vi "Read Measurement.vi"(8 "Error In (no error)":errorcluster, 10 "Value Selection (0: X)":u16(ring) items=["X", "Y", "R [V]", "R [dBm]", "Phi", "CH1 Display", "CH2 Display", "AUX 1", "AUX 2"], 11 "VISA Resource Name":refnum<visa-resource-name>) -> (0 "Error Out":errorcluster, 2 "Value":dbl format="%.2e", 3 "VISA Resource Name Out":refnum<visa-resource-name>)   [LabVIEW 2010, in "Stanford Research 844.lvlib"]
doc: "This VI measures one of parameter's values."
uses:
  <instrlib>/Stanford Research 844/Stanford Research 844.lvlib
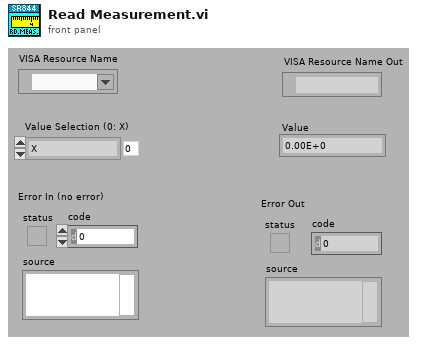
[diagram p1: front panel]
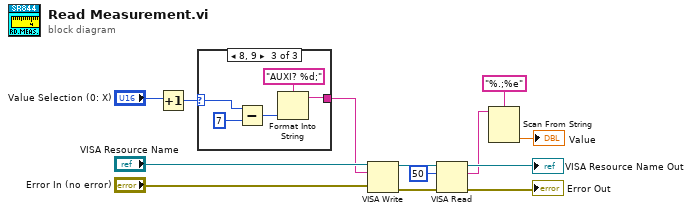
[diagram p0: block diagram]
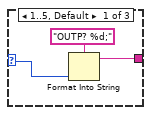
[diagram p2: hidden frame]
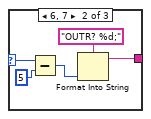
[diagram p3: hidden frame]
diagram:
  n1 = Increment(x="Value Selection (0: X)") -> (x+1=w2:u16)
  n2 = case shown="8, 9" w2 {
    selector: w2 -> [w14 w19 w23]
    tunnel: [w15 w20 w25] -> w1
    frame 1..5, Default {
      n3 = Format Into String(format string="OUTP? %d;", w14) -> (resulting string=w15:string)  [unwired: 2 in, 1 out]
    }
    frame 6, 7 {
      n4 = Subtract(x=w19, y=u16 5) -> (x-y=w17:u16)
      n5 = Format Into String(format string="OUTR? %d;", w17) -> (resulting string=w20:string)  [unwired: 2 in, 1 out]
    }
    frame 8, 9 {
      n6 = Subtract(x=w23, y=u16 7) -> (x-y=w24:u16)
      n7 = Format Into String(format string="AUXI? %d;", w24) -> (resulting string=w25:string)  [unwired: 2 in, 1 out]
    }
  }
  n8 = VISA Write(VISA resource name="VISA Resource Name", write buffer=w1, error in (no error)="Error In (no error)") -> (VISA resource name out=w10:refnum<visa-resource-name>, error out=w9:errorcluster)  [unwired: 1 out]
  n9 = VISA Read(VISA resource name=w10, byte count=u32 50 ("byte count (0)"), error in (no error)=w9) -> (VISA resource name out=→"VISA Resource Name Out":refnum<visa-resource-name>, read buffer=w5:string, error out=→"Error Out":errorcluster)  [unwired: 1 out]
  n10 = Scan From String(format string="%.;%e", input string=w5) -> (output 1=→"Value":dbl)  [unwired: 3 in, 3 out]
